vi "Queues vs Local Variables.vi"() -> ()   [LabVIEW 2012]
panel:
  out "丢失采样":i32
  out "循环速率(ms)":u32
  out "循环速率(ms)":u32
  out "重复采样":i32
  out "采样":i32
  in  "循环速度":u32(ring)=50 items=["等同生产者循环"=50, "最高速度"=0, "2x生产者"=25, "1/2生产者"=100, "1/20生产者"=1000]
  in  "循环速度":u32(ring)=50 items=["等同生产者循环"=50, "最高速度"=0, "2x生产者"=25, "1/2生产者"=100, "1/20生产者"=1000]
  out "队列中采样":i32(slide) scale=0.0..1000.0
  in  "停止":bool
  out "使用局部变量的消费者图表":dbl(graph)
  out "队列消费者图表":dbl(graph)=-9.510565162951542
  out "生产者循环图表":dbl(graph)
  # "生产者循环"
  # "循环时间=50 ms"
  # "使用局部变量的消费者循环"
  # "使用队列的消费者循环"
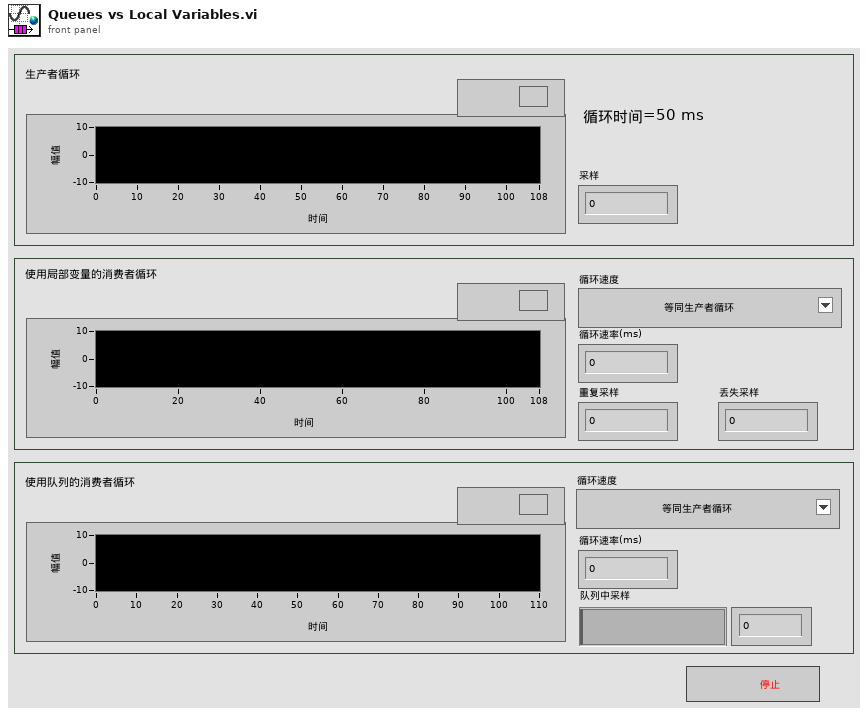
[diagram p1: front panel]
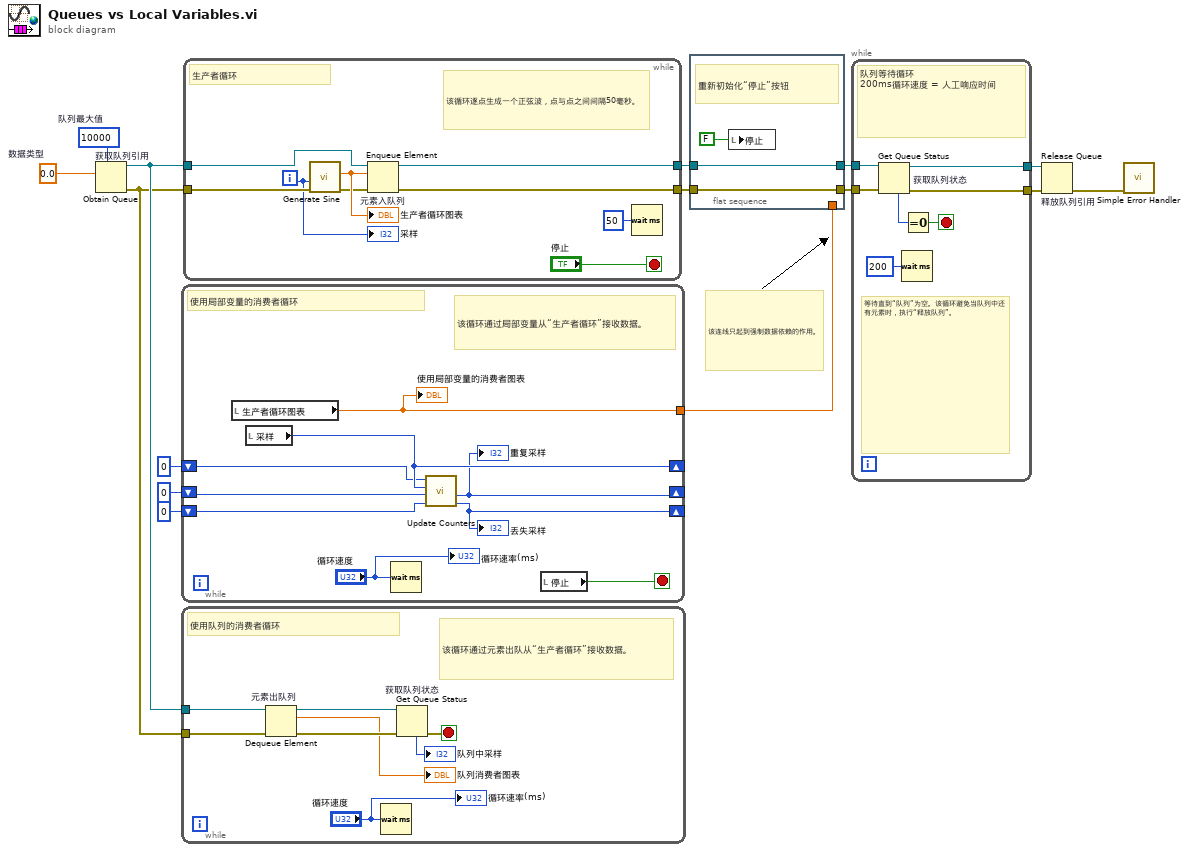
[diagram p0: block diagram]
diagram:
  w1 = 10000  # 队列最大值
  w15 = 0.0  # 数据类型
  # "该连线只起到强制数据依赖的作用。"
  n1 = Obtain Queue "获取队列引用"(max queue size (-1, unlimited)=w1, element data type=w15) -> (queue out=w14:refnum<queue>, error out=w13:errorcluster)  [unwired: 3 in, 1 out]
  n2 = while {
    tunnel: [w23] -> w5
    shift-right: [w21] -> _
    shift-left: 0 ("前一次采样") -> [w20]
    shift-right: [w16] -> _
    shift-left: 0 ("重复") -> [w18]
    shift-right: [w19] -> _
    shift-left: 0 ("丢失") -> [w17]
    stop <- w24 stop-if-true
    # "该循环通过局部变量从“生产者循环”接收数据。"
    # "使用局部变量的消费者循环"
    n3 = local read "生产者循环图表"() -> (w23:dbl)
    "使用局部变量的消费者图表" <- w23
    n4 = local read "采样"() -> (w21:i32)
    n5 = Wait (ms) ("等待(ms)")(milliseconds to wait="循环速度") -> ()  [unwired: 1 out]
    n6 = call "Update Counters.vi"("当前丢失点"=w17, "当前重复点"=w18, "生产者迭代"=w21, "前一个生产者迭代"=w20) -> ("更新的丢失点"=w19:i32, "更新的重复点"=w16:i32)  [unwired: 5 in]
    "重复采样" <- w16
    "丢失采样" <- w19
    n7 = local read "停止"() -> (w24:bool)
    "循环速率(ms)" <- "循环速度"
  }
  n8 = while {
    tunnel: w14 -> [w30]
    tunnel: w13 -> [w29]
    stop <- w27 stop-if-true
    # "该循环通过元素出队从“生产者循环”接收数据。"
    # "使用队列的消费者循环"
    n9 = Dequeue Element "元素出队列"(queue=w30, error in (no error)=w29) -> (queue out=w32:refnum<queue>, element=→"队列消费者图表":dbl, error out=w31:errorcluster)  [unwired: 2 out]
    n10 = Wait (ms) ("等待(ms)")(milliseconds to wait="循环速度") -> ()  [unwired: 1 out]
    n11 = Get Queue Status "获取队列状态"(queue=w32, error in (no error)=w31) -> (error out=w27:errorcluster, # elements in queue=→"队列中采样":i32)  [unwired: 1 in, 6 out]
    "循环速率(ms)" <- "循环速度"
  }
  n12 = while {
    tunnel: w14 -> [w35]
    tunnel: w13 -> [w37]
    tunnel: [w40] -> w8
    tunnel: [w39] -> w7
    i -> [w33]
    stop <- "停止" stop-if-true
    # "该循环逐点生成一个正弦波，点与点之间间隔50毫秒。"
    # "生产者循环"
    n13 = call "Generate Sine.vi"("错误输入"=w37, "数值"=w33) -> ("错误输出"=w36:cluster{"状态":bool, "代码":i32, "源":string}, "正弦波"=w38:dbl)  [unwired: 1 in, 3 out]
    "生产者循环图表" <- w38
    n14 = Enqueue Element "元素入队列"(queue=w35, element=w38, error in (no error)=w36) -> (queue out=w39:refnum<queue>, error out=w40:errorcluster)  [unwired: 2 out]
    n15 = Wait (ms) ("等待(ms)")(milliseconds to wait=u32 50 ("等待时间（毫秒）")) -> ()  [unwired: 1 out]
    "采样" <- w33
  }
  n16 = flat-sequence {
    tunnel: [w44] -> w9
    tunnel: w8 -> [w44]
    tunnel: w7 -> [w43]
    tunnel: [w43] -> w6
    tunnel: w5 -> [_]
    frame #0 {
      # "重新初始化“停止”按钮"
      n17 = local write "停止"(FALSE ("停止")) -> ()
    }
  }
  n18 = while {
    tunnel: w6 -> [w51]
    tunnel: w9 -> [w50]
    tunnel: [w49] -> w12
    tunnel: [w48] -> w11
    stop <- w46 stop-if-true
    # "等待直到“队列”为空。该循环避免当队列中还有元素时，执行“释放队列”。"
    # "队列等待循环\n200ms循环速度 = 人工响应时间"
    n19 = Get Queue Status "获取队列状态"(queue=w51, error in (no error)=w50) -> (queue out=w48:refnum<queue>, error out=w49:errorcluster, # elements in queue=w47:i32)  [unwired: 6 out]
    n20 = Wait (ms) ("等待(ms)")(milliseconds to wait=u32 200 ("等待时间（毫秒）")) -> ()  [unwired: 1 out]
    n21 = Equal To 0? ("等于0？")(x=w47) -> (x = 0?=w46:bool)
  }
  n22 = Release Queue "释放队列引用"(queue=w11, error in (no error)=w12) -> (error out=w10:errorcluster)  [unwired: 3 out]
  n23 = call <vilib>:"Simple Error Handler.vi"("error in (no error)"=w10) -> ()  [unwired: 2 in, 7 out]
